vi "File Controller_Create.vi"(0 "reference in":refnum<class "File Controller.lvclass">, 5 "error in (no error)":errorcluster) -> (14 "reference out":refnum<class "File Controller.lvclass">, 19 "error out":errorcluster)   [LabVIEW 2014, in "File Controller.lvclass"]
doc: "Constructor."
uses:
  File Controller.lvclass
  <vilib>/addons/_AddQ/G#Object/G#Object.lvclass
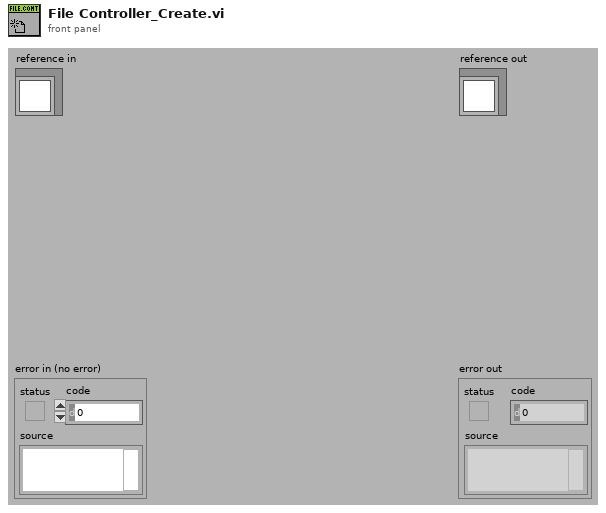
[diagram p1: front panel]
types:
  T1 = typedef "File Controller.lvclass/ClassAttributesRef.ctl" = refnum<data-value>
  T2 = typedef "File Controller.lvclass/ClassAttributes.ctl" = cluster{"Dummy":bool, "File Controller_ref":refnum<class "File Controller.lvclass">}
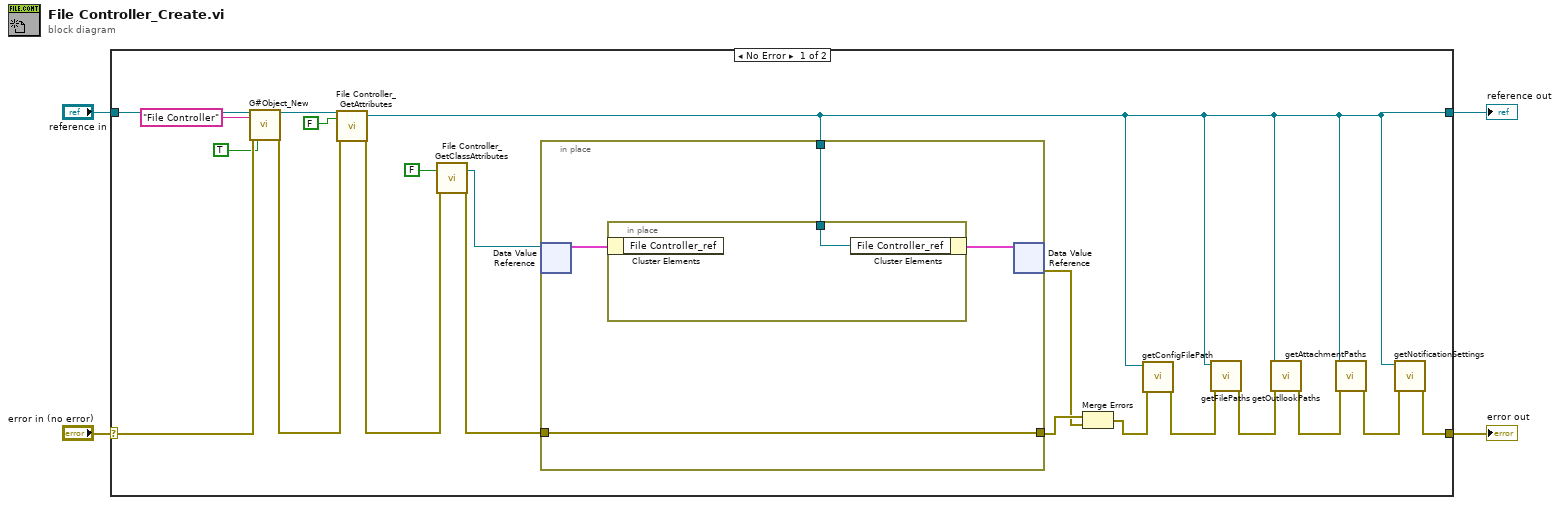
[diagram p0: block diagram]
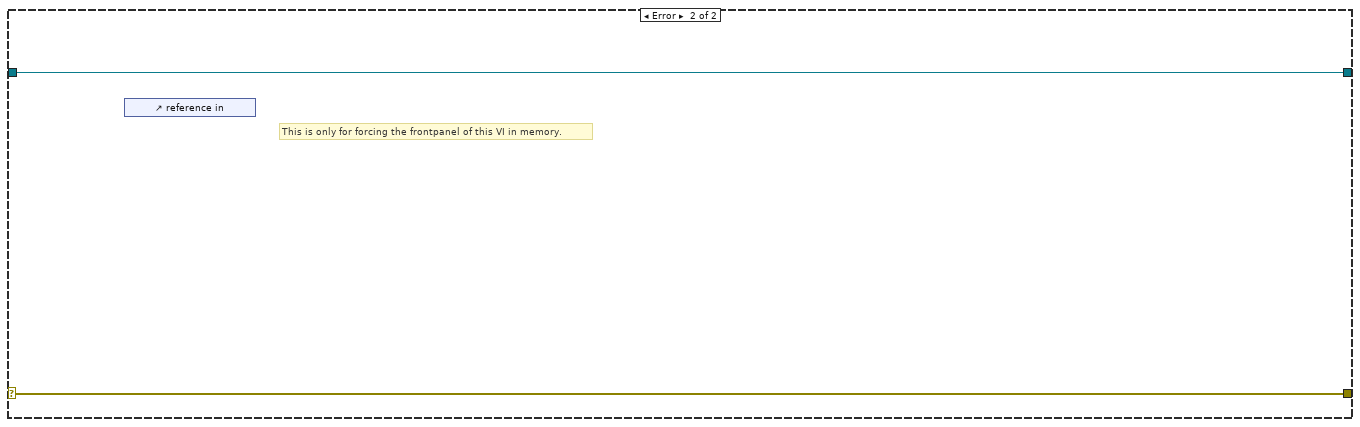
[diagram p2: hidden frame]
diagram:
  n1 = case shown="No Error" "error in (no error)" {
    selector: "error in (no error)" -> [w23 w31]
    tunnel: [w5 w31] -> w3
    tunnel: [w7 w30] -> w1
    tunnel: "reference in" -> [w24 w30]
    frame No Error {
      n2 = call <vilib>:"G#Object_New.vi"("reference in"=w24, "object name"="File Controller", "error in (no error)"=w23, "user counter (T)?"=TRUE ("User Counter")) -> ("reference out"=w19:refnum<class "File Controller.lvclass">, "error out"=w18:errorcluster)  [unwired: 13 in, 1 out]
      n3 = call "File Controller_GetAttributes.vi"("reference in"=w19, "return data? (T)"=FALSE ("return data"), "error in (no error)"=w18) -> ("reference out"=w7:refnum<class "File Controller.lvclass">, "error out"=w16:errorcluster)  [unwired: 13 in, 2 out]
      n4 = call "File Controller_GetClassAttributes.vi"("return data? (T)"=FALSE, "error in (no error)"=w16) -> ("class attributes ref"=w14:T1, "error out"=w15:errorcluster)  [unwired: 14 in, 2 out]
      n5 = in-place {
        in-place-border: w15 -> [w26]
        in-place-border: [w26] -> w21
        in-place-border: w7 -> [w25]
        n6 = in-place-dvr #1(w14) -> (w27:T2)  [unwired: 1 out]
        n7 = in-place {
          in-place-border: w25 -> [w29]
          n8 = in-place-cluster #2(w27) -> ()  [unwired: 1 out]
          n9 = in-place-cluster #2("File Controller_ref"=w29) -> (w28:T2)
        }
        n10 = in-place-dvr #1(w28) -> (w20:errorcluster)  [unwired: 1 out]
      }
      n11 = Merge Errors(w21, w20) -> (w9:errorcluster)
      n12 = call "getConfigFilePath.vi"("error in (no error)"=w9, "reference in"=w7) -> ("error out"=w8:errorcluster)  [unwired: 8 in, 1 out]
      n13 = call "getFilePaths.vi"("error in (no error)"=w8, "reference in"=w7) -> ("error out"=w11:errorcluster)  [unwired: 8 in, 1 out]
      n14 = call "getOutllookPaths.vi"("error in (no error)"=w11, "reference in"=w7) -> ("error out"=w10:errorcluster)  [unwired: 8 in, 1 out]
      n15 = call "getAttachmentPaths.vi"("error in (no error)"=w10, "reference in"=w7) -> ("error out"=w6:errorcluster)  [unwired: 8 in, 1 out]
      n16 = call "getNotificationSettings.vi"("error in (no error)"=w6, "reference in"=w7) -> ("error out"=w5:errorcluster)  [unwired: 8 in, 1 out]
    }
    frame Error {
      # "This is only for forcing the frontpanel of this VI in memory."
      n17 = control-ref of="reference in"() -> ()  [unwired: 1 out]
    }
  }
  "error out" <- w3
  "reference out" <- w1
